vi "weatherapp.vi"() -> ()   [LabVIEW 2022 SP3]
uses:
  <vilib>/Platform/TimedLoop/XDataNode/timing_clust.ctl
  <vilib>/Platform/TimedLoop/XDataNode/nitl_modes.ctl
  <vilib>/Platform/TimedLoop/XDataNode/wakeup.ctl
  <vilib>/httpClient/POSTBuffer.vi
  <vilib>/platform/TimedLoop/XDataNode/XDataNode.xnode
  <vilib>/httpClient/LabVIEWHTTPClient.lvlib
  <vilib>/Platform/TimedLoop/XDataNode/XDNodeRunTimeDep.lvlib
panel:
  in  "stop":bool
  out "JSON string":string
  in  "Cluster":T1 {"temperature" scale=0.0..100.0}
  out "body":string
  out "headers":string
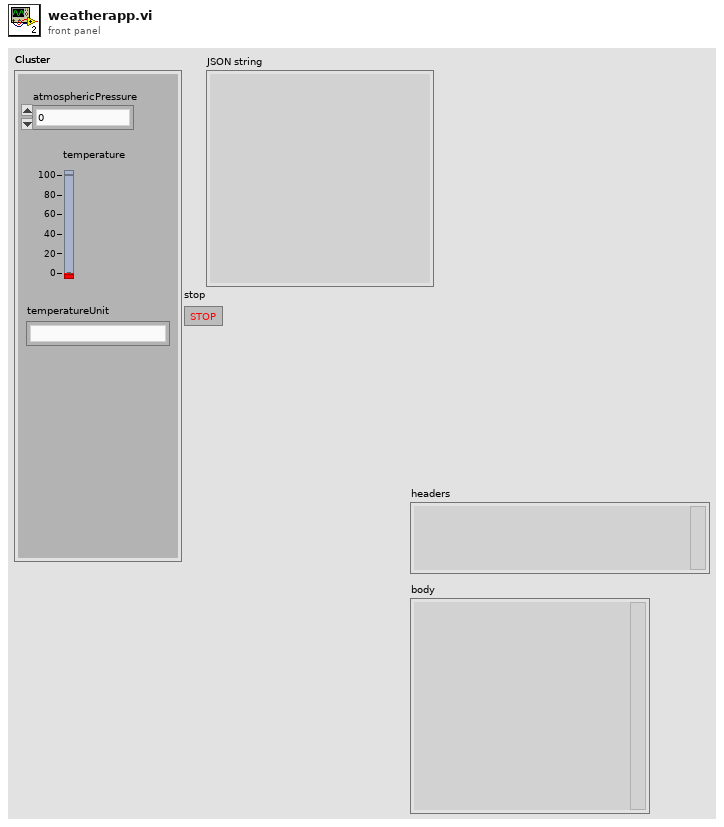
[diagram p1: front panel]
types:
  T1 = cluster{"atmosphericPressure":dbl, "temperature":dbl, "temperatureUnit":string}
  T2 = typedef "XDNodeRunTimeDep.lvlib/timing_clust.ctl" = cluster{"Expected End [f-1]":u64, "Actual End [f-1]":u64, "Finished Late? [f-1]":bool, "Expected End [i-1]":u64, "Actual End [i-1]":u64, "Finished Late? [i-1]":bool, "Expected Start [i]":u64, "Actual Start [i]":u64, "Expected Start [f]":u64, "Actual Start [f]":u64, "Source Name":string, "Structure Name":string, "Period":i64, "Deadline":i64, "Offset":i64, "Start":i64, "Priority":i32, "Timeout":i32, "Mode":T3, "Wakeup Reason":T4, "Error":errorcluster, "Source Type":string, "Secondary Source Type":string, "Global End Time":u64, "Global Start Time":u64, "Frame Duration":u64, "Iteration Duration":u64, "Assigned CPU":i32, "I/O Scan Engine Mode":u32}
  T3 = typedef "XDNodeRunTimeDep.lvlib/nitl_modes.ctl" = enum32{"No Change", "Process missed periods, maintain original phase", "Discard missed periods, maintain original phase", "Process missed periods, ignore original phase", "Discard missed periods, ignore original phase"}
  T4 = typedef "XDNodeRunTimeDep.lvlib/wakeup.ctl" = enum32{"Normal", "Aborted", "Asynchronous wakeup", "Timing source error", "Timed loop error", "Timeout"}
  T5 = typedef "LabVIEWHTTPClient.lvlib/ClientHandle.ctl" = refnum<k1>
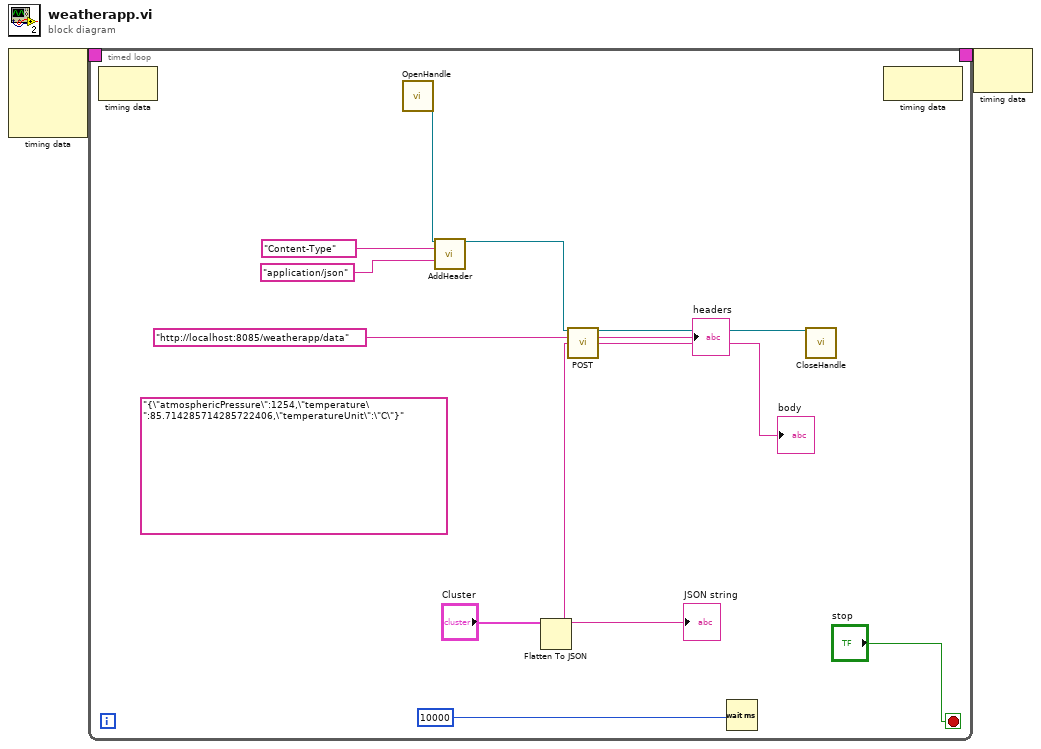
[diagram p0: block diagram]
diagram:
  n1 = node-c288() -> (w2:T2)  [unwired: 4 in]
  n2 = timed-loop {
    timing: w2 -> [_]
    timing-out: [_] -> w1
    stop <- "stop" stop-if-true
    (unwired) "{\"atmosphericPressure\":1254,\"temperature\":85.714285714285722406,\"temperatureUnit\":\"C\"}"
    n3 = node-c288() -> ()  [unwired: 1 in, 1 out]
    n4 = call <vilib>:"OpenHandle.vi"() -> ("client handle out"=w10:T5)  [unwired: 14 in, 1 out]
    n5 = call <vilib>:"AddHeader.vi"("client handle"=w10, "header"="Content-Type", "value"="application/json") -> ("client handle out"=w9:T5)  [unwired: 11 in, 1 out]
    n6 = Flatten To JSON(anything="Cluster") -> (JSON string=w12:string)  [unwired: 2 in, 1 out]
    "JSON string" <- w12
    n7 = call-poly <vilib>:"POST.vi"("client handle"=w9, "url"="http://localhost:8085/weatherapp/data", "buffer"=w12) -> ("client handle out"=w8:T5, "headers"=→"headers":string, "body"=→"body":string)  [unwired: 9 in, 1 out]
    n8 = Wait (ms)(milliseconds to wait=10000) -> ()  [unwired: 1 out]
    n9 = call <vilib>:"CloseHandle.vi"("client handle"=w8) -> ()  [unwired: 14 in, 1 out]
    n10 = node-c288() -> ()  [unwired: 1 in, 1 out]
  }
  n11 = node-c288(w1) -> ()  [unwired: 1 out]
